vi "HT Assign (SubVI).vi"(10 "HT":T2(array[cluster]), 11 "SPINE In":T1) -> (3 "HT Out":T2(array[cluster]))   [LabVIEW 2015]
uses:
  Controls (HOST)/Data to Disk Bundle.ctl
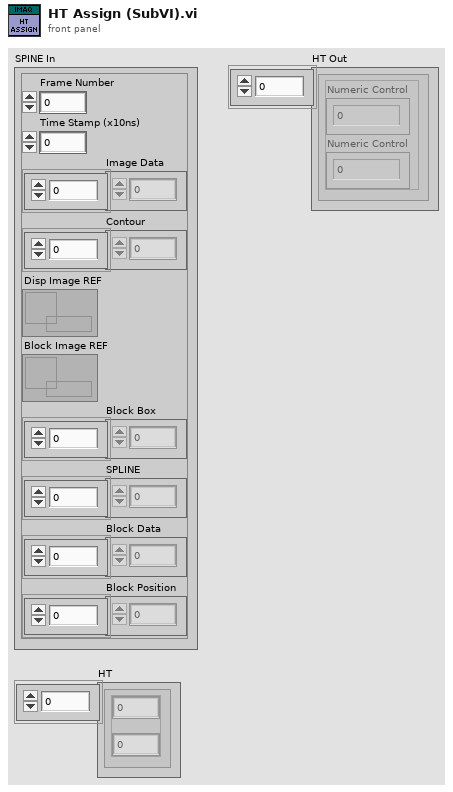
[diagram p1: front panel]
types:
  T1 = typedef "Data to Disk Bundle.ctl" = cluster{"Frame Number":u64, "Time Stamp (x10ns)":u64, "Image Data":u64[], "Contour":u64[], "Disp Image REF":refnum<data-value>, "Block Image REF":refnum<data-value>, "Block Box":u64[], "SPLINE":u64[], "Block Data":u64[], "Block Position":u32[]}
  T2 = cluster{"Numeric Control":i32, "Numeric Control":i32}[]
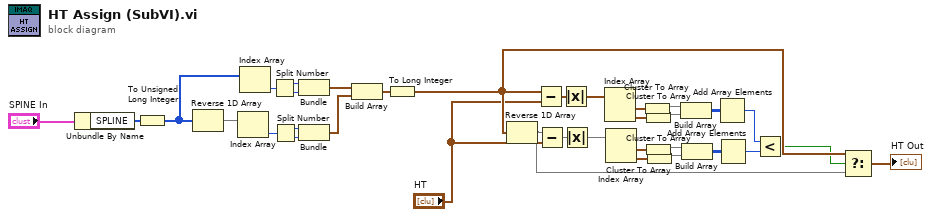
[diagram p0: block diagram]
diagram:
  n1 = Unbundle By Name("SPINE In") -> ("SPLINE"=w21:u64[])
  n2 = To Unsigned Long Integer(number=w21) -> (unsigned 32bit integer=w27:u32[])
  n3 = Reverse 1D Array(array=w27) -> (reversed array=w28:u32[])
  n4 = Index Array(array=w28) -> (element=w24:u32)  [unwired: 1 in]
  n5 = Index Array(array=w27) -> (element=w23:u32)  [unwired: 1 in]
  n6 = Split Number(x=w23) -> (hi(x)=w30:u16, lo(x)=w31:u16)
  n7 = Split Number(x=w24) -> (hi(x)=w25:u16, lo(x)=w26:u16)
  n8 = Bundle(w30, w31) -> (w22:cluster{u16, u16})  [unwired: 1 in]
  n9 = Bundle(w25, w26) -> (w29:cluster{u16, u16})  [unwired: 1 in]
  n10 = Build Array(w22, w29) -> (w32:cluster{u16, u16}[])
  n11 = To Long Integer(number=w32) -> (32bit integer=w33:cluster{i32, i32}[])
  n12 = Reverse 1D Array(array=w33) -> (reversed array=w18:cluster{i32, i32}[])
  n13 = Subtract(x=w33, y="HT") -> (x-y=w2:cluster{i32, i32}[])
  n14 = Subtract(x=w18, y="HT") -> (x-y=w16:cluster{i32, i32}[])
  n15 = Absolute Value(x=w2) -> (abs(x)=w3:cluster{i32, i32}[])
  n16 = Absolute Value(x=w16) -> (abs(x)=w15:cluster{i32, i32}[])
  n17 = Index Array(array=w3) -> (element #1=w4:cluster{i32, i32}, element #2=w5:cluster{i32, i32})  [unwired: 2 in]
  n18 = Index Array(array=w15) -> (element #1=w14:cluster{i32, i32}, element #2=w13:cluster{i32, i32})  [unwired: 2 in]
  n19 = Cluster To Array(cluster=w4) -> (array=w6:i32[])
  n20 = Cluster To Array(cluster=w5) -> (array=w7:i32[])
  n21 = Cluster To Array(cluster=w14) -> (array=w12:i32[])
  n22 = Cluster To Array(cluster=w13) -> (array=w11:i32[])
  n23 = Build Array(w6, w7) -> (w8:i32[][])
  n24 = Build Array(w12, w11) -> (w10:i32[][])
  n25 = Add Array Elements(numeric array=w8) -> (sum=w9:i32)
  n26 = Add Array Elements(numeric array=w10) -> (sum=w17:i32)
  n27 = Less?(x=w9, y=w17) -> (x < y?=w19:bool)
  n28 = Select(t=w33, s=w19, f=w18) -> (s? t:f=→"HT Out":cluster{i32, i32}[])
